vi "send_image.vi"(7 "force sending?":bool, 8 "error in (no error)":errorcluster, 9 "image finished?":bool=TRUE, 10 "image (channels)":refnum<class "Image.lvclass">[](array[class]), 11 "DisplayDL090216 in":refnum<class "DisplayDL090216.lvclass">) -> (0 "error out":errorcluster, 3 "DisplayDL090216 out":refnum<class "DisplayDL090216.lvclass">, 4 "# elements in queue":i32)   [LabVIEW 2010, in "DisplayDL090216.lvclass"]
uses:
  DisplayDL090216.lvclass
  common/classes/Image/Image/Image.lvclass
  DisplayDL090216.lvclass/DisplayDL090216.ctl
  GenericDisplay/GenericDisplay/GenericDisplay.lvclass
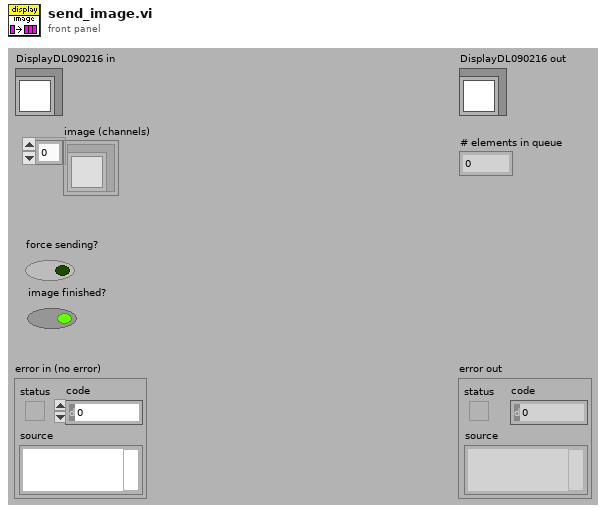
[diagram p1: front panel]
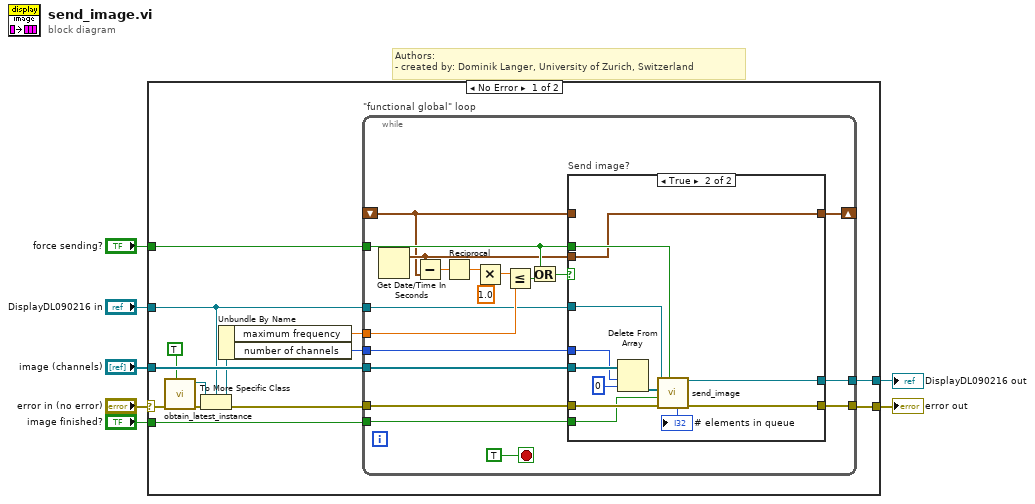
[diagram p0: block diagram]
diagram:
  # "Authors: \n- created by: Dominik Langer, University of Zurich, Switzerland"
  n1 = case shown="No Error" "error in (no error)" {
    selector: "error in (no error)" -> [w16 w57]
    tunnel: [w20 w57] -> w2
    tunnel: "force sending?" -> [w19 _]
    tunnel: "DisplayDL090216 in" -> [w15 w56]
    tunnel: [w18 w56] -> w1
    tunnel: "image (channels)" -> [w17 _]
    tunnel: "image finished?" -> [w21 _]
    frame No Error {
      n2 = call "obtain_latest_instance.vi"("quick, but maybe outdated?"=TRUE, "error in (no error)"=w16) -> ("error out"=w11:errorcluster, "GenericDisplay out"=w10:refnum<class "GenericDisplay.lvclass">)  [unwired: 8 in]
      n3 = To More Specific Class(target class=w15, reference=w10, error in=w11) -> (specific class reference=w14:refnum<class "DisplayDL090216.lvclass">, error out=w13:errorcluster)
      n4 = Unbundle By Name(w14) -> ("maximum frequency"=w8:dbl[unit], "number of channels"=w9:i32)
      n5 = while "\"functional global\" loop" {
        tunnel: w8 -> [w37]
        tunnel: w13 -> [w35]
        tunnel: w21 -> [w33]
        tunnel: [w32] -> w20
        tunnel: w19 -> [w31]
        tunnel: w15 -> [w30]
        tunnel: [w29] -> w18
        tunnel: w17 -> [w28]
        tunnel: w9 -> [w27]
        shift-right: [w24] -> _
        shift-left: _ -> [w23]
        stop <- TRUE stop-if-true
        n6 = Get Date/Time In Seconds() -> (seconds since 1Jan1904=w25:timestamp)
        n7 = Subtract(x=w25, y=w23) -> (x-y=w40:dbl)
        n8 = Reciprocal(x=w40) -> (1/x=w38:dbl)
        n9 = Multiply(x=w38, y=dbl[unit] 1.0) -> (x*y=w22:dbl[unit])
        n10 = Less Or Equal?(x=w22, y=w37) -> (x <= y?=w36:bool)
        n11 = Or(x=w31, y=w36) -> (x .or. y?=w34:bool)
        n12 = case "Send image?" shown="True" w34 {
          tunnel: w35 -> [w43 w54]
          tunnel: w33 -> [_ w51]
          tunnel: [w43 w52] -> w32
          tunnel: w31 -> [_ w50]
          tunnel: w30 -> [w42 w49]
          tunnel: [w42 w48] -> w29
          tunnel: w28 -> [_ w47]
          tunnel: w27 -> [_ w46]
          tunnel: w25 -> [_ w44]
          tunnel: [w41 w44] -> w24
          tunnel: w23 -> [w41 _]
          frame False {
          }
          frame True {
            n13 = Delete From Array(array=w47, length=w46, index=0) -> (deleted portion=w45:refnum<class "Image.lvclass">[])  [unwired: 1 out]
            n14 = call-parent "send_image.vi"("force sending?"=w50, "error in (no error)"=w54, "image finished?"=w51, "image (channels)"=w45, "GenericToplevelComponent in"=w49) -> ("error out"=w52:errorcluster, "GenericToplevelComponent out"=w48:refnum<class "DisplayDL090216.lvclass">, "# elements in queue"=→"# elements in queue":i32)  [unwired: 4 in]
          }
        }
      }
    }
    frame Error {
    }
  }
  "error out" <- w2
  "DisplayDL090216 out" <- w1
